vi "gpanel_generate_ui_events.vi"(8 "error in (no error)":errorcluster, 11 "galvo_panel in":refnum<class "galvo_panel.lvclass">) -> (0 "error out":errorcluster, 2 "ui_events":T1, 3 "galvo_panel out":refnum<class "galvo_panel.lvclass">)   [LabVIEW 2015, in "galvo_panel.lvclass"]
uses:
  galvo_panel.lvclass
  galvo_event_refs.ctl
  galvo_ui_events.ctl
  galvo_panel.lvclass/galvo_panel.ctl
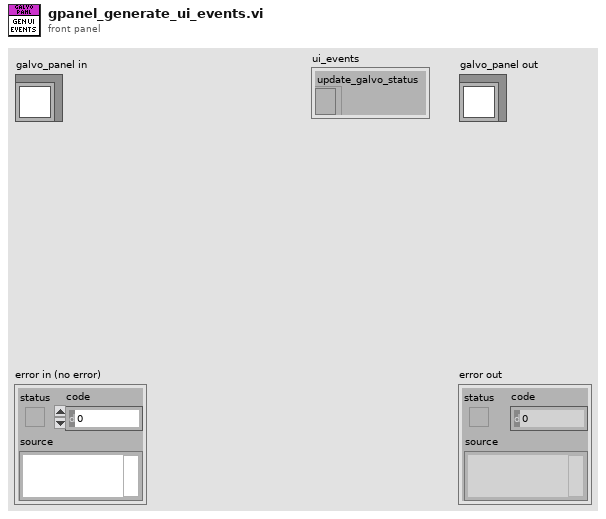
[diagram p1: front panel]
types:
  T1 = typedef "galvo_event_refs.ctl" = cluster{"update_galvo_status":refnum<event-registration>}
  T2 = typedef "galvo_ui_events.ctl" = cluster{"update_galvo_status":refnum<user-event>}
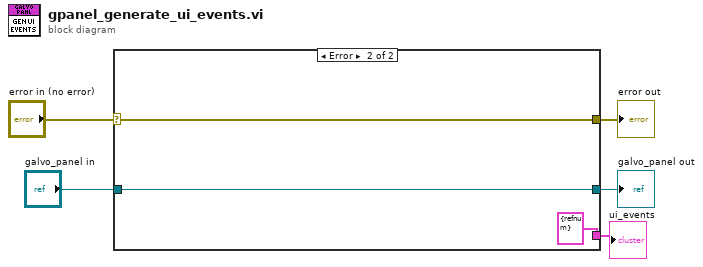
[diagram p0: block diagram]
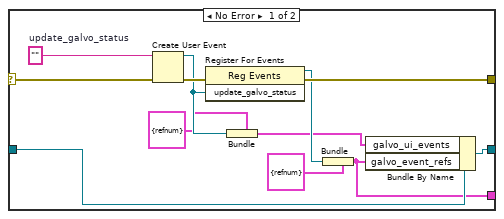
[diagram p2: hidden frame]
diagram:
  n1 = case shown="Error" "error in (no error)" {
    selector: "error in (no error)" -> [w15 w20]
    tunnel: [w14 w20] -> w4
    tunnel: [w7 w19] -> w2
    tunnel: "galvo_panel in" -> [w9 w19]
    tunnel: [w6 T1 {"update_galvo_status"=refnum} ("output cluster")] -> w1
    frame No Error {
      w17 = ""  # update_galvo_status
      n2 = Create User Event(user event datatype=w17, error in=w15) -> (user event=w11:refnum<user-event>, error out=w16:errorcluster)
      n3 = register-events(error in=w16, w11) -> (reference out=w13:refnum<event-registration>, error out=w14:errorcluster)  [unwired: 1 in]
      n4 = Bundle(cluster=T2 {"update_galvo_status"=refnum} ("output cluster"), "update_galvo_status"=w11) -> (w8:T2)
      n5 = Bundle(cluster=T1 {"update_galvo_status"=refnum} ("output cluster"), "update_galvo_status"=w13) -> (w6:T1)
      n6 = Bundle By Name(cluster=w9, "galvo_ui_events"=w8, "galvo_event_refs"=w6) -> (w7:refnum<class "galvo_panel.lvclass">)
    }
    frame Error {
    }
  }
  "error out" <- w4
  "galvo_panel out" <- w2
  "ui_events" <- w1
